vi "Serialization Test.vi"() -> ()   [LabVIEW 2019]
uses:
  <vilib>/gpm_packages/@cs/lookup-table/Source/LookupTable/LookupTable.lvclass/LookupTable.ctl
  689a59ec-a001-42b7-ae47-e45672baa5f0.vi
  1c837f5e-d41a-4954-8212-f9e446fdb006.vi
  12776c44-63e3-45c8-a9f0-cdbf5d5ca944.vi
  05c712d3-ba66-4d68-8b40-a383c1921b55.vi
  930595ed-04bd-4994-abc5-ece6fc73146a.vi
  16fc5843-f95b-4bc5-bfb3-73bfc2cdd38d.vi
  6956caf3-d76c-450f-a123-7a39bbbbf995.vi
  <vilib>/gpm_packages/@cs/lookup-table/Source/LookupTable/Read Table Reference.vi
  689a59ec-a001-42b7-ae47-e45672baa5f0.vi/dcd00a04-2c4e-4e1a-8d84-0c914a50e7e2.vi
  1c837f5e-d41a-4954-8212-f9e446fdb006.vi/ccc500d2-507e-4ff5-b27d-bb6f4b13a422.vi
  12776c44-63e3-45c8-a9f0-cdbf5d5ca944.vi/f9a8bb6f-8849-4c76-9092-8d3e86669fd8.vi
  05c712d3-ba66-4d68-8b40-a383c1921b55.vi/3cd82fc8-dc00-4933-b61c-67407f2b8898.vi
  16fc5843-f95b-4bc5-bfb3-73bfc2cdd38d.vi/a5d07c9e-2b31-4e1d-9f14-c9f2b11c7bf8.vi
  6956caf3-d76c-450f-a123-7a39bbbbf995.vi/8daa45f2-c7e2-49e9-8fa8-02cb14f947f0.vi
  <vilib>/gpm_packages/@cs/variant/Source/Scalar Data to String.vi
  <vilib>/Utility/Data Type/Get Type Information.vi
  <vilib>/Utility/Data Type/Get Refnum Information.vi
  <vilib>/gpm_packages/@cs/lookup-table/Source/LookupTable/LookupTable.lvclass
  <vilib>/gpm_packages/@cs/variant/Source/VariantExtensions.lvlib
panel:
  out "Values":variant[](array[variant])
  out "Value as String":string
  out "Type Name":string
  out "value":variant
  out "Value 2":i32
  out "data string":string
  out "Value":i32
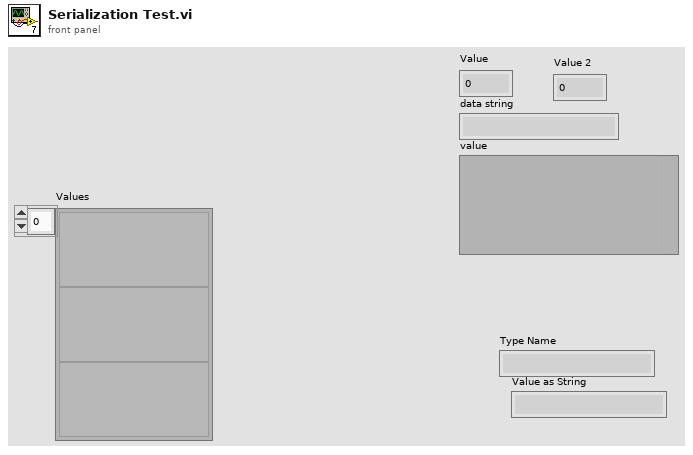
[diagram p1: front panel]
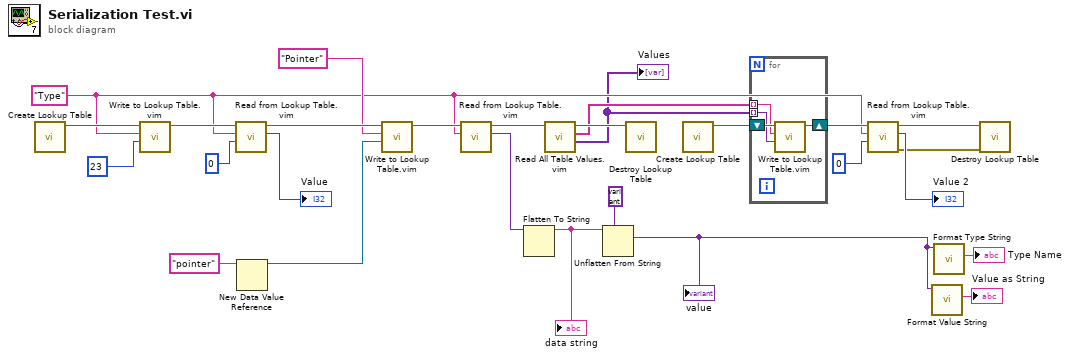
[diagram p0: block diagram]
diagram:
  w5 = "Type" ("Item Name")
  n1 = call <vilib>:"Create Lookup Table.vi"() -> ("LookupTable Reference"=w25:refnum<data-value>)  [unwired: 10 in, 1 out]
  n2 = call "Write to Lookup Table.vim"("Item"=23, "Item Name"=w5, "LookupTable Reference"=w25) -> ("LookupTable Reference Out"=w22:refnum<data-value>)  [unwired: 6 in, 2 out]
  n3 = call "Read from Lookup Table.vim"("Type"=0, "Item Name"=w5, "LookupTable Reference"=w22) -> ("Value"=→"Value":i32, "LookupTable Reference Out"=w9:refnum<data-value>)  [unwired: 5 in, 2 out]
  n4 = New Data Value Reference(data value="pointer") -> (data value reference=w7:refnum<data-value>)  [unwired: 1 in, 1 out]
  n5 = call "Write to Lookup Table.vim"("Item"=w7, "Item Name"="Pointer", "LookupTable Reference"=w9) -> ("LookupTable Reference Out"=w8:refnum<data-value>)  [unwired: 6 in, 2 out]
  n6 = call "Read from Lookup Table.vim"("Item Name"=w5, "LookupTable Reference"=w8) -> ("Value"=w23:variant, "LookupTable Reference Out"=w4:refnum<data-value>)  [unwired: 6 in, 2 out]
  n7 = Flatten To String(anything=w23) -> (data string=w27:string)  [unwired: 3 in, 2 out]
  "data string" <- w27
  n8 = call "Read All Table Values.vim"("LookupTable Reference"=w4) -> ("Values"=w1:variant[], "Names"=w2:string[], "LookupTable Reference Out"=w3:refnum<data-value>)  [unwired: 7 in, 1 out]
  "Values" <- w1
  n9 = Unflatten From String(type=variant ("variant"), binary string=w27) -> (value=w12:variant)  [unwired: 3 in, 2 out]
  "value" <- w12
  n10 = call <vilib>:"Destroy Lookup Table.vi"("LookupTable Reference"=w3) -> ()  [unwired: 10 in, 1 out]
  n11 = call <vilib>:"Create Lookup Table.vi"() -> ("LookupTable Reference"=w14:refnum<data-value>)  [unwired: 10 in, 1 out]
  n12 = for {
    shift-right: [w31] -> w19
    shift-left: w14 -> [w30]
    tunnel: w2 -> [w29] mode=indexing
    tunnel: w1 -> [w28] mode=indexing
    n13 = call "Write to Lookup Table.vim"("Item"=w28, "Item Name"=w29, "LookupTable Reference"=w30) -> ("LookupTable Reference Out"=w31:refnum<data-value>)  [unwired: 6 in, 2 out]
  }
  n14 = call "Read from Lookup Table.vim"("Type"=0, "Item Name"=w5, "LookupTable Reference"=w19) -> ("error out"=w15:errorcluster, "Value"=→"Value 2":i32, "LookupTable Reference Out"=w16:refnum<data-value>)  [unwired: 5 in, 1 out]
  n15 = call <vilib>:"Format Value String.vi"("Data"=w12) -> ("Value as String"=→"Value as String":string)  [unwired: 9 in, 1 out]
  n16 = call <vilib>:"Format Type String.vi"("Data Type"=w12) -> ("Type Name"=→"Type Name":string)  [unwired: 9 in, 1 out]
  n17 = call <vilib>:"Destroy Lookup Table.vi"("error in (no error)"=w15, "LookupTable Reference"=w16) -> ()  [unwired: 9 in, 1 out]
